vi "GOMDBTS2048 get Peak.vi"(8 "error in (no error)":errorcluster, 11 "handle":i32) -> (0 "error out":errorcluster, 1 "function return":i32, 2 "power":dbl, 3 "lambda":dbl)   [LabVIEW 2015, in "GOMDBTS2048.lvlib"]
doc: "GOBTS2048DLL int __stdcall GOMDBTS2048_getPeak(int handle, double *lambda, double *power);"
uses:
  GOMDBTS2048.lvlib
  runtime/GOMDBTS2048.dll
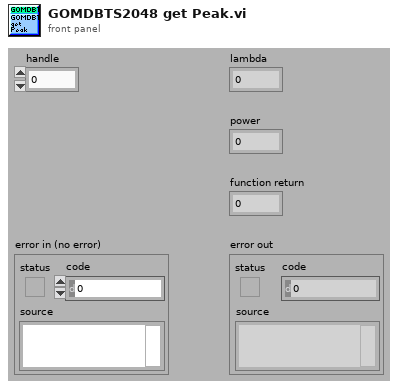
[diagram p1: front panel]
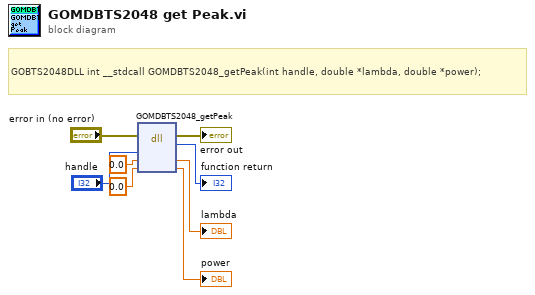
[diagram p0: block diagram]
diagram:
  # "GOBTS2048DLL int __stdcall GOMDBTS2048_getPeak(int handle, double *lambda, double *power);"
  n1 = dll-call lib="C:/Users/rkoch/Documents/GO_Library/runtime/GOMDBTS2048.*" fn="GOMDBTS2048_getPeak"(error in="error in (no error)", "handle"="handle", "lambda"=0.0, "power"=0.0) -> (error out=→"error out":errorcluster, →"function return":i32, "lambda"=→"lambda":dbl, "power"=→"power":dbl)  [unwired: 3 in, 1 out]
